vi "Mean Values-P_1.vi"() -> ()   [LabVIEW 2010]
uses:
  <vilib>/measure/madcrms.llb/Basic Averaged DC-RMS for 1 Chan.vi
  <vilib>/measure/NI_MAPro.lvlib
panel:
  in  "Calculate Background?":bool
  in  "Trim? (FALSE CAN BREAK MEMORY ON 9K+)":bool
  out "size(s)":i32
  in  "Modify Path?":bool
  out "Mod Length #Samples":dbl
  in  "Mod Duration S":dbl=0.3
  out "Trigger Index":dbl
  in  "Total Length (S)":i32=2
  in  "Pretrigger Duration%":i32=10
  in  "sample rate Recorder":i32=16384
  in  "Icai Start value \n(S after trigger mod starts)":dbl=0.05
  out "Waveform Graph":waveform(dbl)(graph)
  out "Noise Ground":dbl format="%0.2p"
  out "Vpp Factor":dbl
  in  "Vpp":dbl=1.38
  out "sensitivity factor":dbl
  in  "Lock-In Sens in mv":dbl=10.0
  out "appended path":path
  in  "search string":string
  out "name":string
  in  "path":path
  in  "#Files to read":i32
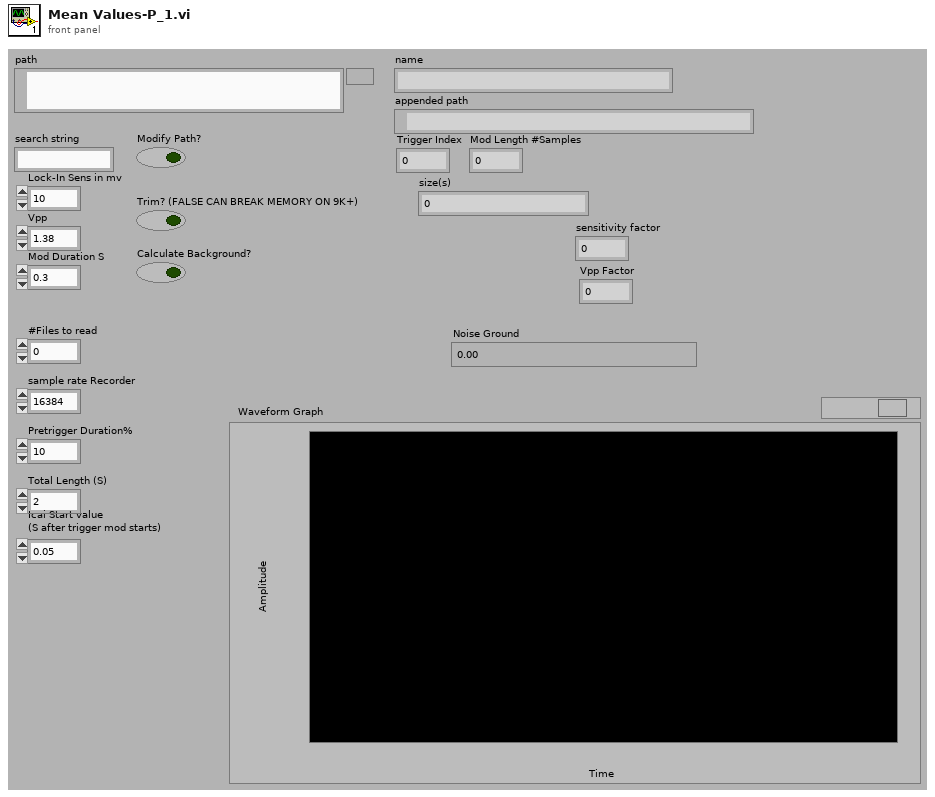
[diagram p1: front panel]
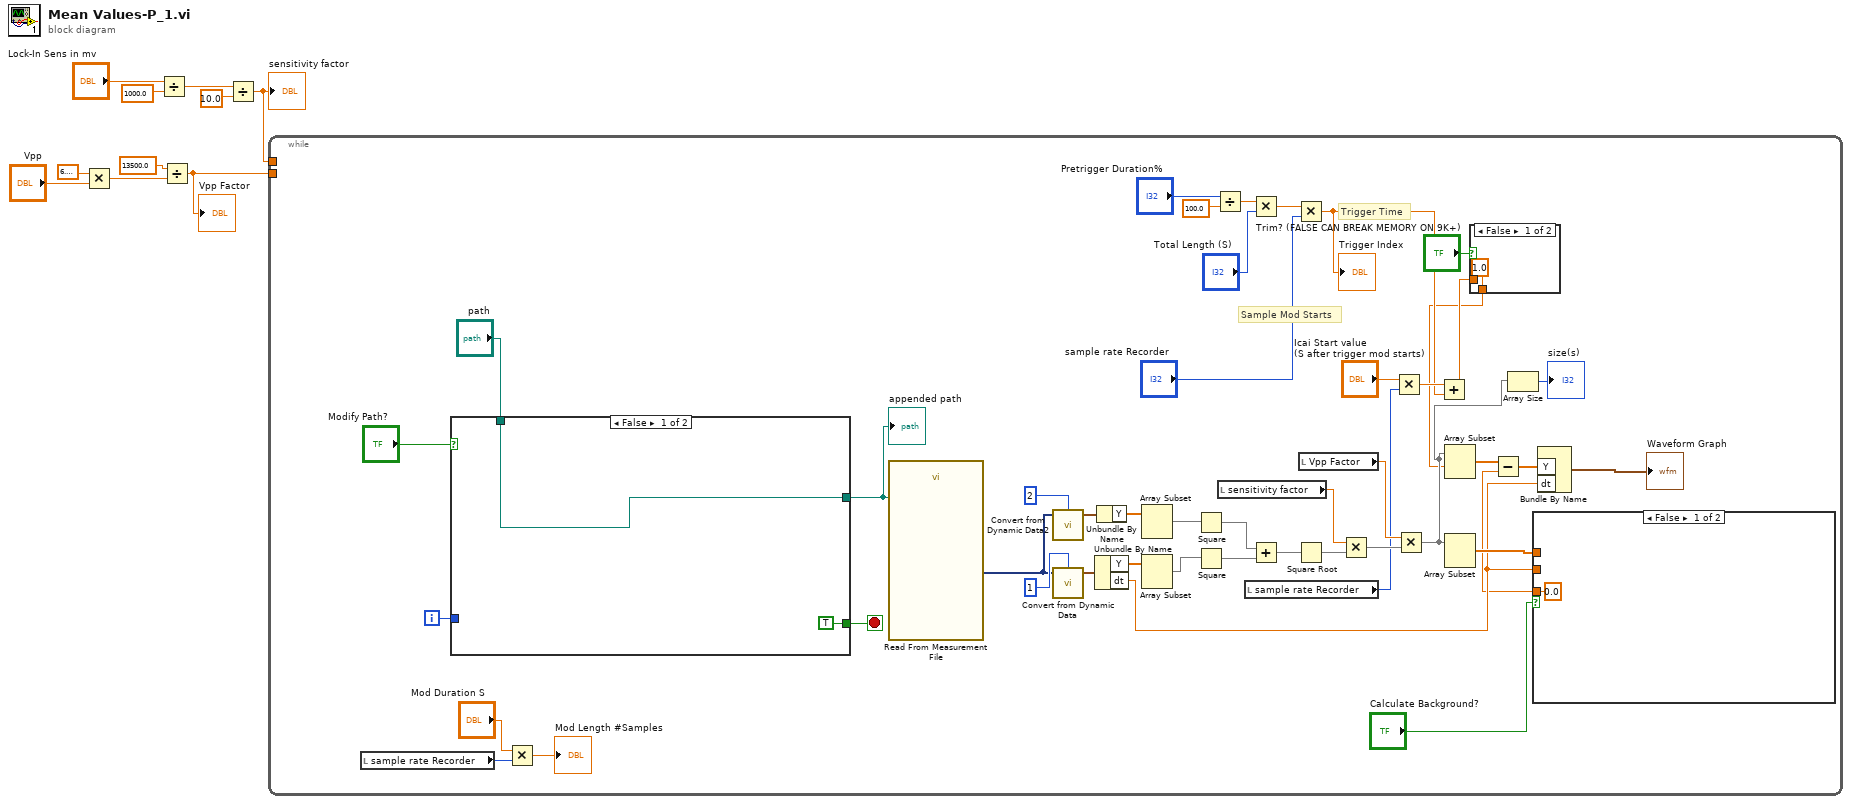
[diagram p0: block diagram]
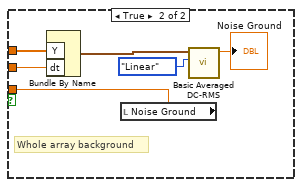
[diagram p2: hidden frame]
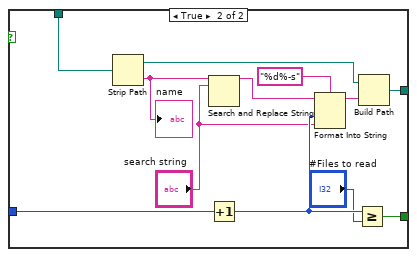
[diagram p4: hidden frame]
diagram:
  n1 = Multiply(x=6.283185307179586, y="Vpp") -> (x*y=w9:dbl)
  n2 = Divide(x="Lock-In Sens in mv", y=1000.0) -> (x/y=w5:dbl)
  n3 = Divide(x=13500.0, y=w9) -> (x/y=w1:dbl)
  "Vpp Factor" <- w1
  n4 = Divide(x=w5, y=10.0) -> (x/y=w2:dbl)
  "sensitivity factor" <- w2
  n5 = while {
    tunnel: w2 -> [_]
    tunnel: w1 -> [_]
    i -> [w20]
    stop <- w21 stop-if-true
    # "Sample Mod Starts"
    # "Trigger Time"
    n6 = local read "sample rate Recorder"() -> (w28:i32)
    n7 = case shown="False" "Modify Path?" {
      tunnel: [TRUE w71] -> w21
      tunnel: w20 -> [_ w70]
      tunnel: [w66 w69] -> w19
      tunnel: "path" -> [w66 w68]
      frame False {
      }
      frame True {
        n8 = Strip Path(path=w68) -> (stripped path=w78:path, name=w73:string)
        "name" <- w73
        n9 = Search and Replace String(input string=w73, search string="search string") -> (result string=w74:string)  [unwired: 6 in, 3 out]
        n10 = Increment(x=w70) -> (x+1=w79:i32)
        n11 = Format Into String(format string="%d%-s", initial string=w74, w79, "search string") -> (resulting string=w77:string)  [unwired: 1 in, 1 out]
        n12 = Greater Or Equal?(x=w79, y="#Files to read") -> (x >= y?=w71:bool)
        n13 = Build Path(base path=w78, name or relative path=w77) -> (appended path=w69:path)
      }
    }
    "appended path" <- w19
    n14 = Multiply(x="Mod Duration S", y=w28) -> (x*y=→"Mod Length #Samples":dbl)
    n15 = call "Read From Measurement File"("Filename"=w19) -> ("Signals"=w55:dynamicdata)  [unwired: 5 in, 5 out]
    n16 = call "Convert from Dynamic Data2"("Dynamic Data Type"=w55, "Channel"=2) -> ("Waveform"=w50:waveform(dbl))  [unwired: 2 in]
    n17 = call "Convert from Dynamic Data"("Dynamic Data Type"=w55, "Channel"=1) -> ("Waveform"=w53:waveform(dbl))  [unwired: 2 in]
    n18 = Unbundle By Name(w53) -> ("Y"=w52:dbl[], "dt"=w38:dbl)
    n19 = Unbundle By Name(w50) -> ("Y"=w51:dbl[])
    n20 = Array Subset(array=w51) -> (w45:dbl[])  [unwired: 2 in]
    n21 = Array Subset(array=w52) -> (w41:dbl[])  [unwired: 2 in]
    n22 = Square(x=w45) -> (x^2=w48:dbl[])
    n23 = Square(x=w41) -> (x^2=w47:dbl[])
    n24 = Divide(x="Pretrigger Duration%", y=100.0) -> (x/y=w33:dbl)
    n25 = local read "sensitivity factor"() -> (w44:dbl)
    n26 = local read "sample rate Recorder"() -> (w30:i32)
    n27 = Multiply(x=w33, y="Total Length (S)") -> (x*y=w29:dbl)
    n28 = Add(x=w48, y=w47) -> (x+y=w49:dbl[])
    n29 = Multiply(x=w29, y="sample rate Recorder") -> (x*y=w23:dbl)
    "Trigger Index" <- w23
    n30 = Square Root(x=w49) -> (sqrt(x)=w40:dbl[])
    n31 = local read "Vpp Factor"() -> (w43:dbl)
    n32 = Multiply(x=w44, y=w40) -> (x*y=w42:dbl[])
    n33 = Multiply(x="Icai Start value \n(S after trigger mod starts)", y=w30) -> (x*y=w25:dbl)
    n34 = Multiply(x=w43, y=w42) -> (x*y=w18:dbl[])
    n35 = Add(x=w25, y=w23) -> (x+y=w14:dbl)
    n36 = Array Subset(array=w18) -> (w46:dbl[])  [unwired: 2 in]
    n37 = case shown="False" "Trim? (FALSE CAN BREAK MEMORY ON 9K+)" {
      tunnel: w14 -> [_ w65]
      tunnel: [1.0 w65] -> w13
      frame False {
      }
      frame True {
      }
    }
    n38 = Array Subset(array=w18, index=w13) -> (w37:dbl[])  [unwired: 1 in]
    n39 = Array Size(array=w18) -> (size(s)=→"size(s)":i32)
    n40 = case shown="False" "Calculate Background?" {
      tunnel: w46 -> [_ w61]
      tunnel: w38 -> [_ w59]
      tunnel: [0.0 ("Noise Ground") w58] -> w11
      frame False {
      }
      frame True {
        # "Whole array background"
        n41 = Bundle By Name("Y"=w61, "dt"=w59) -> (w62:waveform(dbl))  [unwired: 1 in]
        n42 = local read "Noise Ground"() -> (w58:dbl)
        n43 = call-poly <vilib>:"Basic Averaged DC-RMS.vi"("averaging type"=enum16{"Linear", "Exponential"}."Linear", "signal in"=w62) -> ("DC value"=→"Noise Ground":dbl)  [unwired: 6 in, 3 out]
      }
    }
    n44 = Subtract(x=w37, y=w11) -> (x-y=w36:dbl[])
    n45 = Bundle By Name("Y"=w36, "dt"=w38) -> (→"Waveform Graph":waveform(dbl))  [unwired: 1 in]
  }
